vi "Actor Core.vi"(8 "error in":errorcluster, 11 "Setting View in":refnum<class "Setting View.lvclass">) -> (0 "error out":errorcluster, 3 "Actor out":refnum<class "Actor.lvclass">)   [LabVIEW 2020, in "[V]Setting View.lvlib" / "Setting View.lvclass"]
doc: "(<B>Filename</B>: Actor Framework.lvlib:Actor.lvclass:Actor Core.vi)\n\nReceives messages to the actor, reacts to them, and initiates any error handling that may shut the actor down.\n\nDescendant classes may override this VI to append parallel tasks for the actor to complete while it handles messages. Overrides use the Call Parent Class Method node."
uses:
  Setting View.lvclass
  C:/Program Files (x86)/National Instruments/LabVIEW 2020/vi.lib/ActorFramework/Actor/Actor.lvclass
  <vilib>/ActorFramework/Actor/Actor.lvclass
  Setting View.lvclass/Setting View.ctl
  Depden On/Abstruct View/Abstruct View/Abstruct View.lvclass/Abstruct View.ctl
  <vilib>/ActorFramework/Actor/Actor.lvclass/Actor.ctl
  <vilib>/ActorFramework/Message Enqueuer/Message Enqueuer.lvclass/Message Enqueuer.ctl
  Color Interface/Color/Color Message.lvclass
  Color Interface/Color/Color Message.lvclass/Color Message.ctl
  Color Interface/Color Interface Messages/Set Color Msg/Set Color Msg.lvclass/Set Color Msg.ctl
  Color Interface/Color/Accessors/Write BG Color.vi
  Color Interface/Color/Accessors/Write Fornt Color.vi
  Depden On/Abstruct View/Abstruct View/Data Accessors/Read Stop Event.vi
  Depden On/Abstruct View/Abstruct View/Data Accessors/Write FP.Title.vi
  Depden On/Abstruct View/Abstruct View/Data Accessors/Write Core VI.vi
  <vilib>/ActorFramework/Message Enqueuer/Init from Existing Queue.vi
  <vilib>/ActorFramework/Message Enqueuer/Enqueue.vi
  <vilib>/ActorFramework/Stop Msg/Stop Msg.lvclass
  C:/Program Files (x86)/National Instruments/LabVIEW 2020/vi.lib/ActorFramework/Message/Message.lvclass
  Color Interface/Color Interface Messages/Set Color Msg/Set Color Msg.lvclass
  Setting View Messages/Set Color To Caller Msg/Set Color To Caller Msg.lvclass
  <vilib>/ActorFramework/Message Priority Queue/Priority Enqueue.vi
  Depden On/MVVM Framework/MVVM Abstruct View/MVVM Abstruct View/MVVM Abstruct View.lvclass
  <vilib>/ActorFramework/Message Enqueuer/Message Enqueuer.lvclass
panel:
  out "Black":bool
  out "Green":bool
  out "BLUE":bool
  in  "Cancel":bool
  in  "OK":bool
  # "Theme"
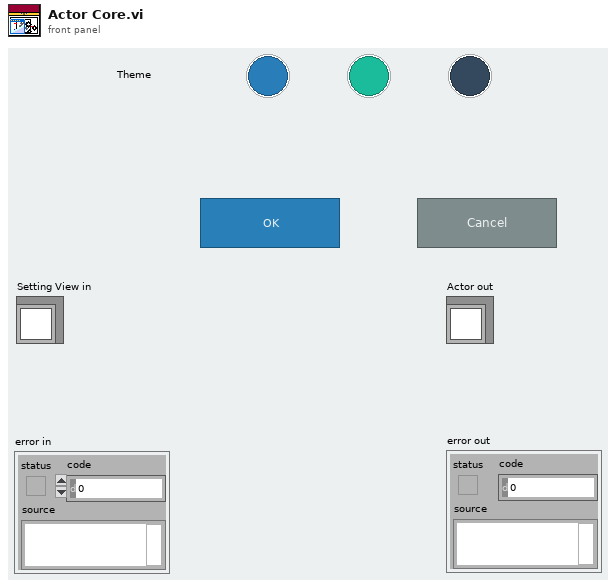
[diagram p1: front panel]
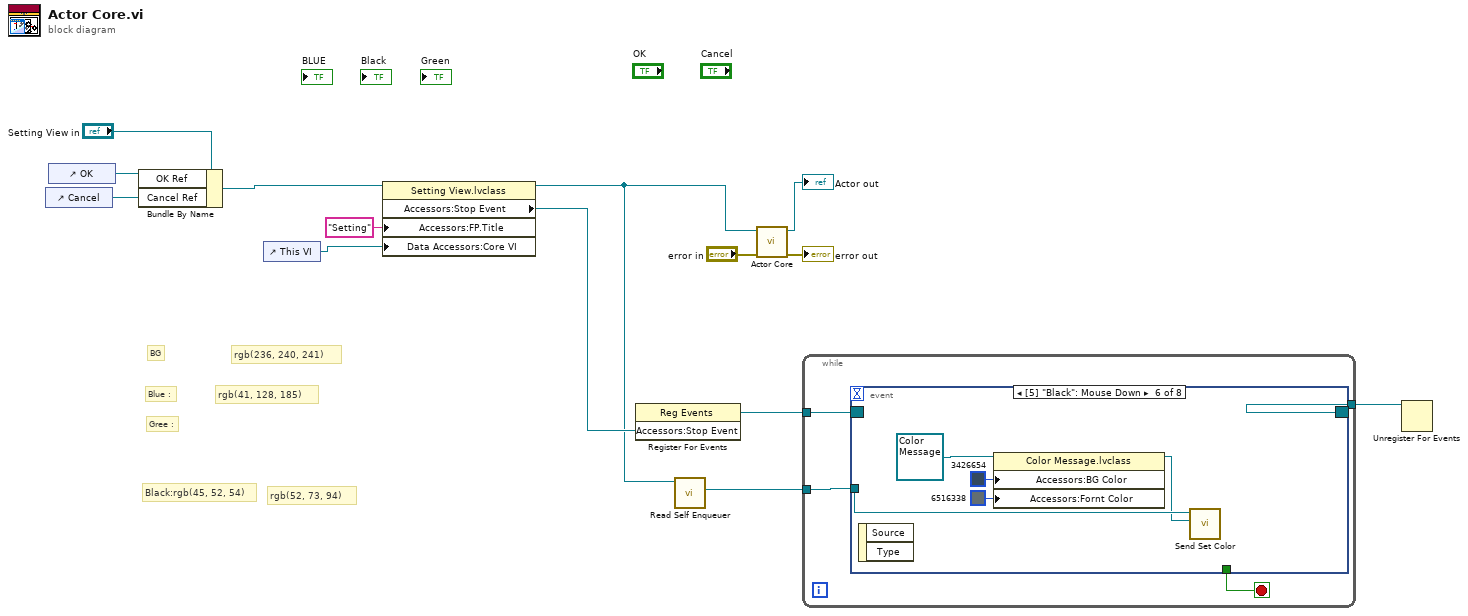
[diagram p0: block diagram]
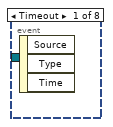
[diagram p2: hidden frame]
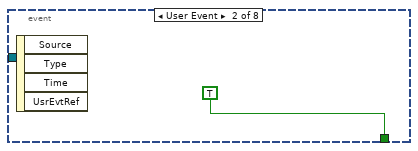
[diagram p3: hidden frame]
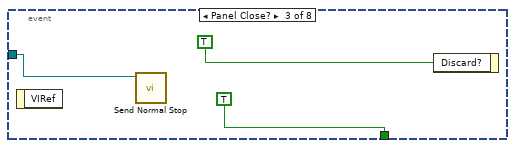
[diagram p4: hidden frame]
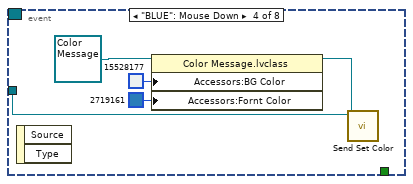
[diagram p5: hidden frame]
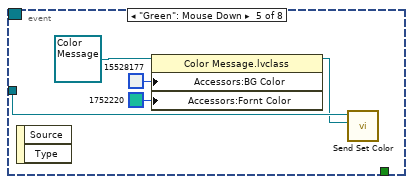
[diagram p6: hidden frame]
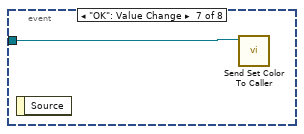
[diagram p7: hidden frame]
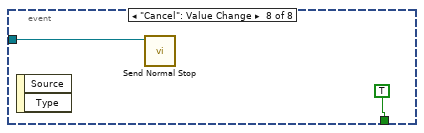
[diagram p8: hidden frame]
diagram:
  # "rgb(236, 240, 241)"
  # "BG"
  # "rgb(52, 73, 94)"
  # "Black:rgb(45, 52, 54)"
  # "Gree :"
  # "rgb(41, 128, 185)"
  # "Blue :"
  n1 = control-ref of="Cancel"() -> (w2:refnum<vi>)
  n2 = control-ref of="OK"() -> (w3:refnum<vi>)
  n3 = Bundle By Name(cluster="Setting View in", "OK Ref"=w3, "Cancel Ref"=w2) -> (w1:refnum<class "Setting View.lvclass">)
  n4 = control-ref of="This VI"() -> (w5:refnum<vi>)
  n5 = property class="Setting View.lvclass"(reference=w1, "Accessors:FP.Title"="Setting" ("FP.Title"), "Data Accessors:Core VI"=w5) -> (reference out=w7:refnum<class "Setting View.lvclass">, "Accessors:Stop Event"=w11:refnum<user-event>)  [unwired: 1 in, 1 out]
  n6 = register-events(w11) -> (reference out=w10:refnum<event-registration>)  [unwired: 2 in, 1 out]
  n7 = call <vilib>:"Read Self Enqueuer.vi"("Actor"=w7) -> ("Self Enqueuer"=w8:refnum<class "Message Enqueuer.lvclass">)  [unwired: 10 in]
  n8 = call-parent "Actor Core.vi"("error in"="error in", "Abstruct View in"=w7) -> ("error out"=→"error out":errorcluster, "Actor out"=→"Actor out":refnum<class "Actor.lvclass">)  [unwired: 8 in]
  n9 = while {
    tunnel: w10 -> [w18]
    tunnel: [w17] -> w9
    tunnel: w8 -> [w15]
    stop <- w16 stop-if-true
    n10 = event shown="[5] \"Black\": Mouse Down" {
      selector: w18 -> [_ _ _ _ _ _ _ _]
      dyn-events: [_ _ _ _ _ _ _ _] -> w17
      timeout: _ -> [_ _ _ _ _ _ _ _]
      tunnel: [_ TRUE TRUE _ _ _ _ TRUE] -> w16
      tunnel: w15 -> [_ _ w21 w27 w32 w37 w38 w39]
      event Timeout {
        n11 = event-data() -> ()  [unwired: 1 in, 3 out]
      }
      event User Event {
        n12 = event-data() -> ()  [unwired: 1 in, 4 out]
      }
      event Panel Close? {
        n13 = event-data() -> ()  [unwired: 1 in, 1 out]
        n14 = call <vilib>:"Send Normal Stop.vi"("Message Enqueuer"=w21) -> ()  [unwired: 10 in, 1 out]
        n15 = event-data("Discard?"=TRUE) -> ()  [unwired: 1 in, 1 out]
      }
      event "BLUE": Mouse Down {
        n16 = event-data() -> ()  [unwired: 1 in, 2 out]
        n17 = property class="Color Message.lvclass"(reference=refnum<class "Color Message.lvclass"> refnum ("Color Message.lvclass"), "Accessors:BG Color"=u32 15528177 ("BG Color"), "Accessors:Fornt Color"=u32 2719161 ("Fornt Color")) -> (reference out=w25:refnum<class "Color Message.lvclass">)  [unwired: 1 in, 1 out]
        n18 = call "Send Set Color.vi"("Color Message.lvclass"=w25, "Message Enqueuer"=w27) -> ()  [unwired: 8 in, 2 out]
      }
      event "Green": Mouse Down {
        n19 = event-data() -> ()  [unwired: 1 in, 2 out]
        n20 = property class="Color Message.lvclass"(reference=refnum<class "Color Message.lvclass"> refnum ("Color Message.lvclass"), "Accessors:BG Color"=u32 15528177 ("BG Color"), "Accessors:Fornt Color"=u32 1752220 ("Fornt Color")) -> (reference out=w30:refnum<class "Color Message.lvclass">)  [unwired: 1 in, 1 out]
        n21 = call "Send Set Color.vi"("Color Message.lvclass"=w30, "Message Enqueuer"=w32) -> ()  [unwired: 8 in, 2 out]
      }
      event "Black": Mouse Down {
        n22 = event-data() -> ()  [unwired: 1 in, 2 out]
        n23 = property class="Color Message.lvclass"(reference=refnum<class "Color Message.lvclass"> refnum ("Color Message.lvclass"), "Accessors:BG Color"=u32 3426654 ("BG Color"), "Accessors:Fornt Color"=u32 6516338 ("Fornt Color")) -> (reference out=w35:refnum<class "Color Message.lvclass">)  [unwired: 1 in, 1 out]
        n24 = call "Send Set Color.vi"("Color Message.lvclass"=w35, "Message Enqueuer"=w37) -> ()  [unwired: 8 in, 2 out]
      }
      event "OK": Value Change {
        n25 = event-data() -> ()  [unwired: 1 in, 1 out]
        n26 = call "Send Set Color To Caller.vi"("Message Enqueuer"=w38) -> ()  [unwired: 9 in, 2 out]
      }
      event "Cancel": Value Change {
        n27 = event-data() -> ()  [unwired: 1 in, 2 out]
        n28 = call <vilib>:"Send Normal Stop.vi"("Message Enqueuer"=w39) -> ()  [unwired: 10 in, 1 out]
      }
    }
  }
  n29 = Unregister For Events(event registration refnum=w9) -> ()  [unwired: 1 in, 1 out]
